vi "Initialize.vi"(8 "error in (no error)":errorcluster, 10 "Serial Port":string, 11 "Serial Device in":refnum<class "Serial Device.lvclass">) -> (0 "error out":errorcluster, 3 "Serial Device out":refnum<class "Serial Device.lvclass">)   [LabVIEW 2017, in "Serial Device.lvclass"]
uses:
  Serial Device.lvclass
  Serial Device.lvclass/Serial Device.ctl
  Set Serial Port.vi
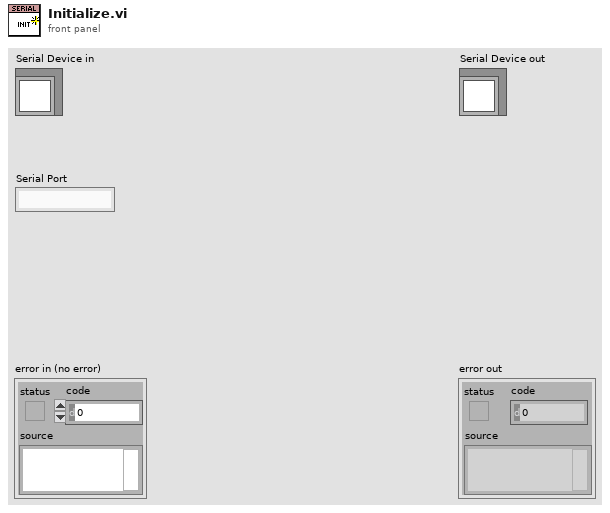
[diagram p1: front panel]
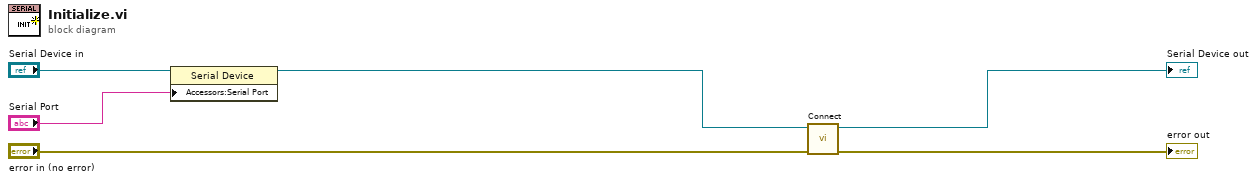
[diagram p0: block diagram]
diagram:
  n1 = property class="Serial Device"(reference="Serial Device in", "Accessors:Serial Port"="Serial Port") -> (reference out=w2:refnum<class "Serial Device.lvclass">)  [unwired: 1 in, 1 out]
  n2 = call-dynamic "Connect.vi"("error in (no error)"="error in (no error)", "Serial Device in"=w2) -> ("error out"=→"error out":errorcluster, "Serial Device out"=→"Serial Device out":refnum<class "Serial Device.lvclass">)  [unwired: 8 in]
